vi "PumpValveHeater.vi"() -> ()   [LabVIEW 2015]
uses:
  PumpValve.ctl
  <vilib>/DAQmx/write.llb/DAQmx Write (Digital 1D Bool NChan 1Samp 1Line).vi
  <vilib>/DAQmx/miscellaneous.llb/DAQmx Fill In Error Info.vi
  <vilib>/addons/control/pid/pid.llb/PID (DBL).vi
  <vilib>/addons/control/pid/NI_PID_pid.lvlib
panel:
  out "Numeric 2":dbl
  out "Numeric":dbl
  out "Heater On/off":bool
  out "Meter (Temp Sensor)":dbl(knob) scale=0.0..10.0
  in  "Stop Maintaining Temp":bool
  in  "PID gains Temp":T1={"proportional gain (Kc)"=1.0, "integral time (Ti, min)"=0.01, "derivative time (Td, min)"=0.0} {"derivative time (Td, min)" format="%.3f"; "integral time (Ti, min)" format="%.3f"; "proportional gain (Kc)" format="%.3f"}
  in  "Temp Setting":dbl
  in  "Maintain Temp":bool
  in  "Stop Maintaining Pressure":bool
  in  "PID gains":T1={"proportional gain (Kc)"=1.0, "integral time (Ti, min)"=0.01, "derivative time (Td, min)"=0.0} {"derivative time (Td, min)" format="%.3f"; "integral time (Ti, min)" format="%.3f"; "proportional gain (Kc)" format="%.3f"}
  out "Meter (Pressure Sensor)":dbl(knob) scale=0.0..10.0
  in  "Pressure Setting":dbl
  in  "Maintain pressure":bool
  in  "On/Off Temp":bool
  in  "Manual Mode Temp":bool
  in  "stop controller":bool
  in  "Duty cycle % (0-100)":dbl=50.0
  in  "stop PWM":bool
  in  "Steps in a cycle":i32=256
  in  "Cycle time (s)":dbl=5.0
  in  "On/Off (Pump)":bool
  in  "Open/Close (Blue)":bool
  in  "Open/Close (Green)":bool
  in  "Manual Mode Pump/Valve":bool
  out "Invalid fill%":bool
  out "Tank":u32(slide) scale=0.0..100.0
  in  "Drain %":u32
  in  "Fill %":u32
  in  "Drain":bool
  in  "Stop Program":bool
  in  "Fill":bool
  # "Temp only adjusts up (do nothing to cool?)"
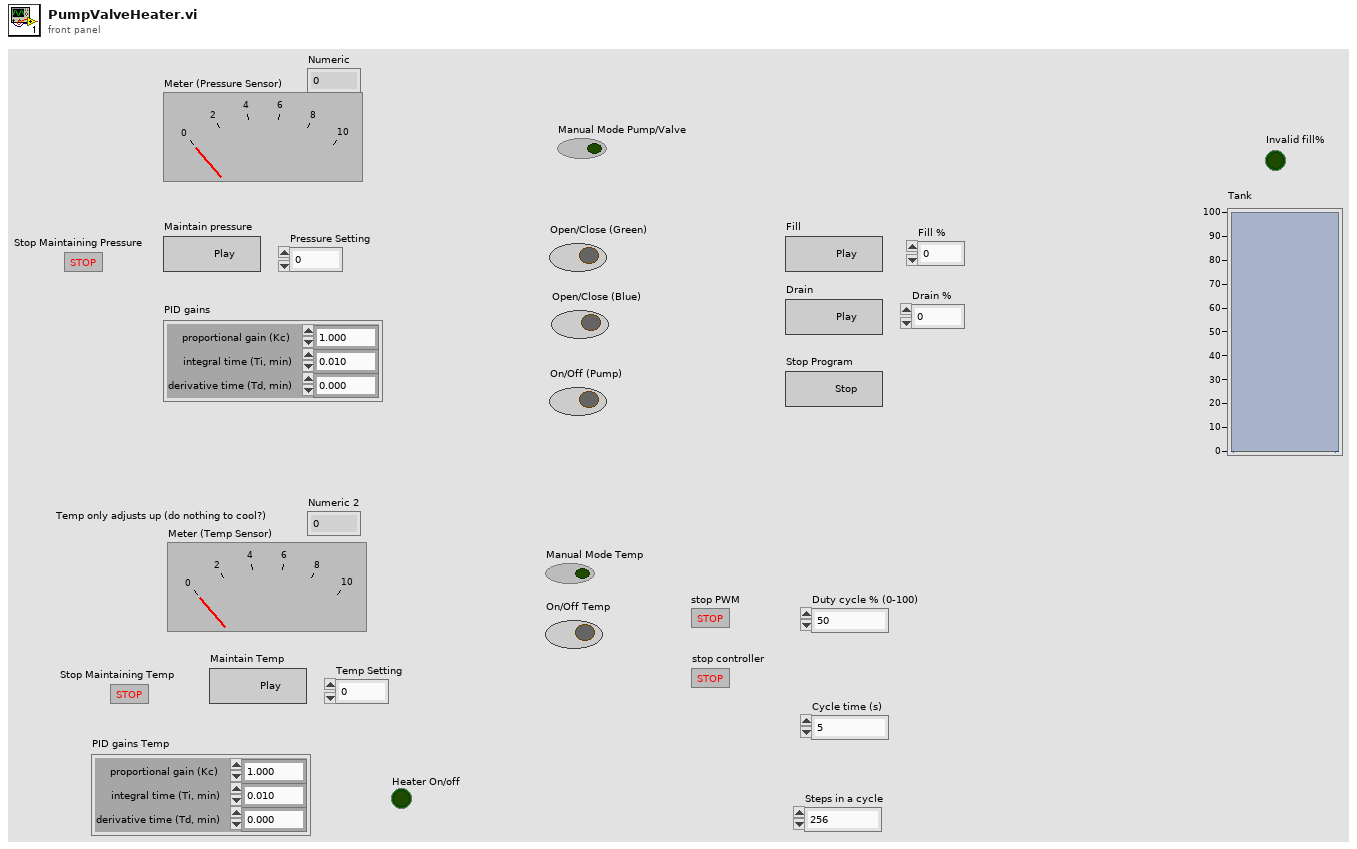
[diagram p1: front panel]
types:
  T1 = cluster{"proportional gain (Kc)":dbl, "integral time (Ti, min)":dbl, "derivative time (Td, min)":dbl}
  T2 = typedef "PumpValve.ctl" = enum16{"PressureSetting", "ManualPressure", "ManualTemp", "Idle Temp", "Set Temp", "Initialize", "Idle", "Fill", "Drain", "Stop"}
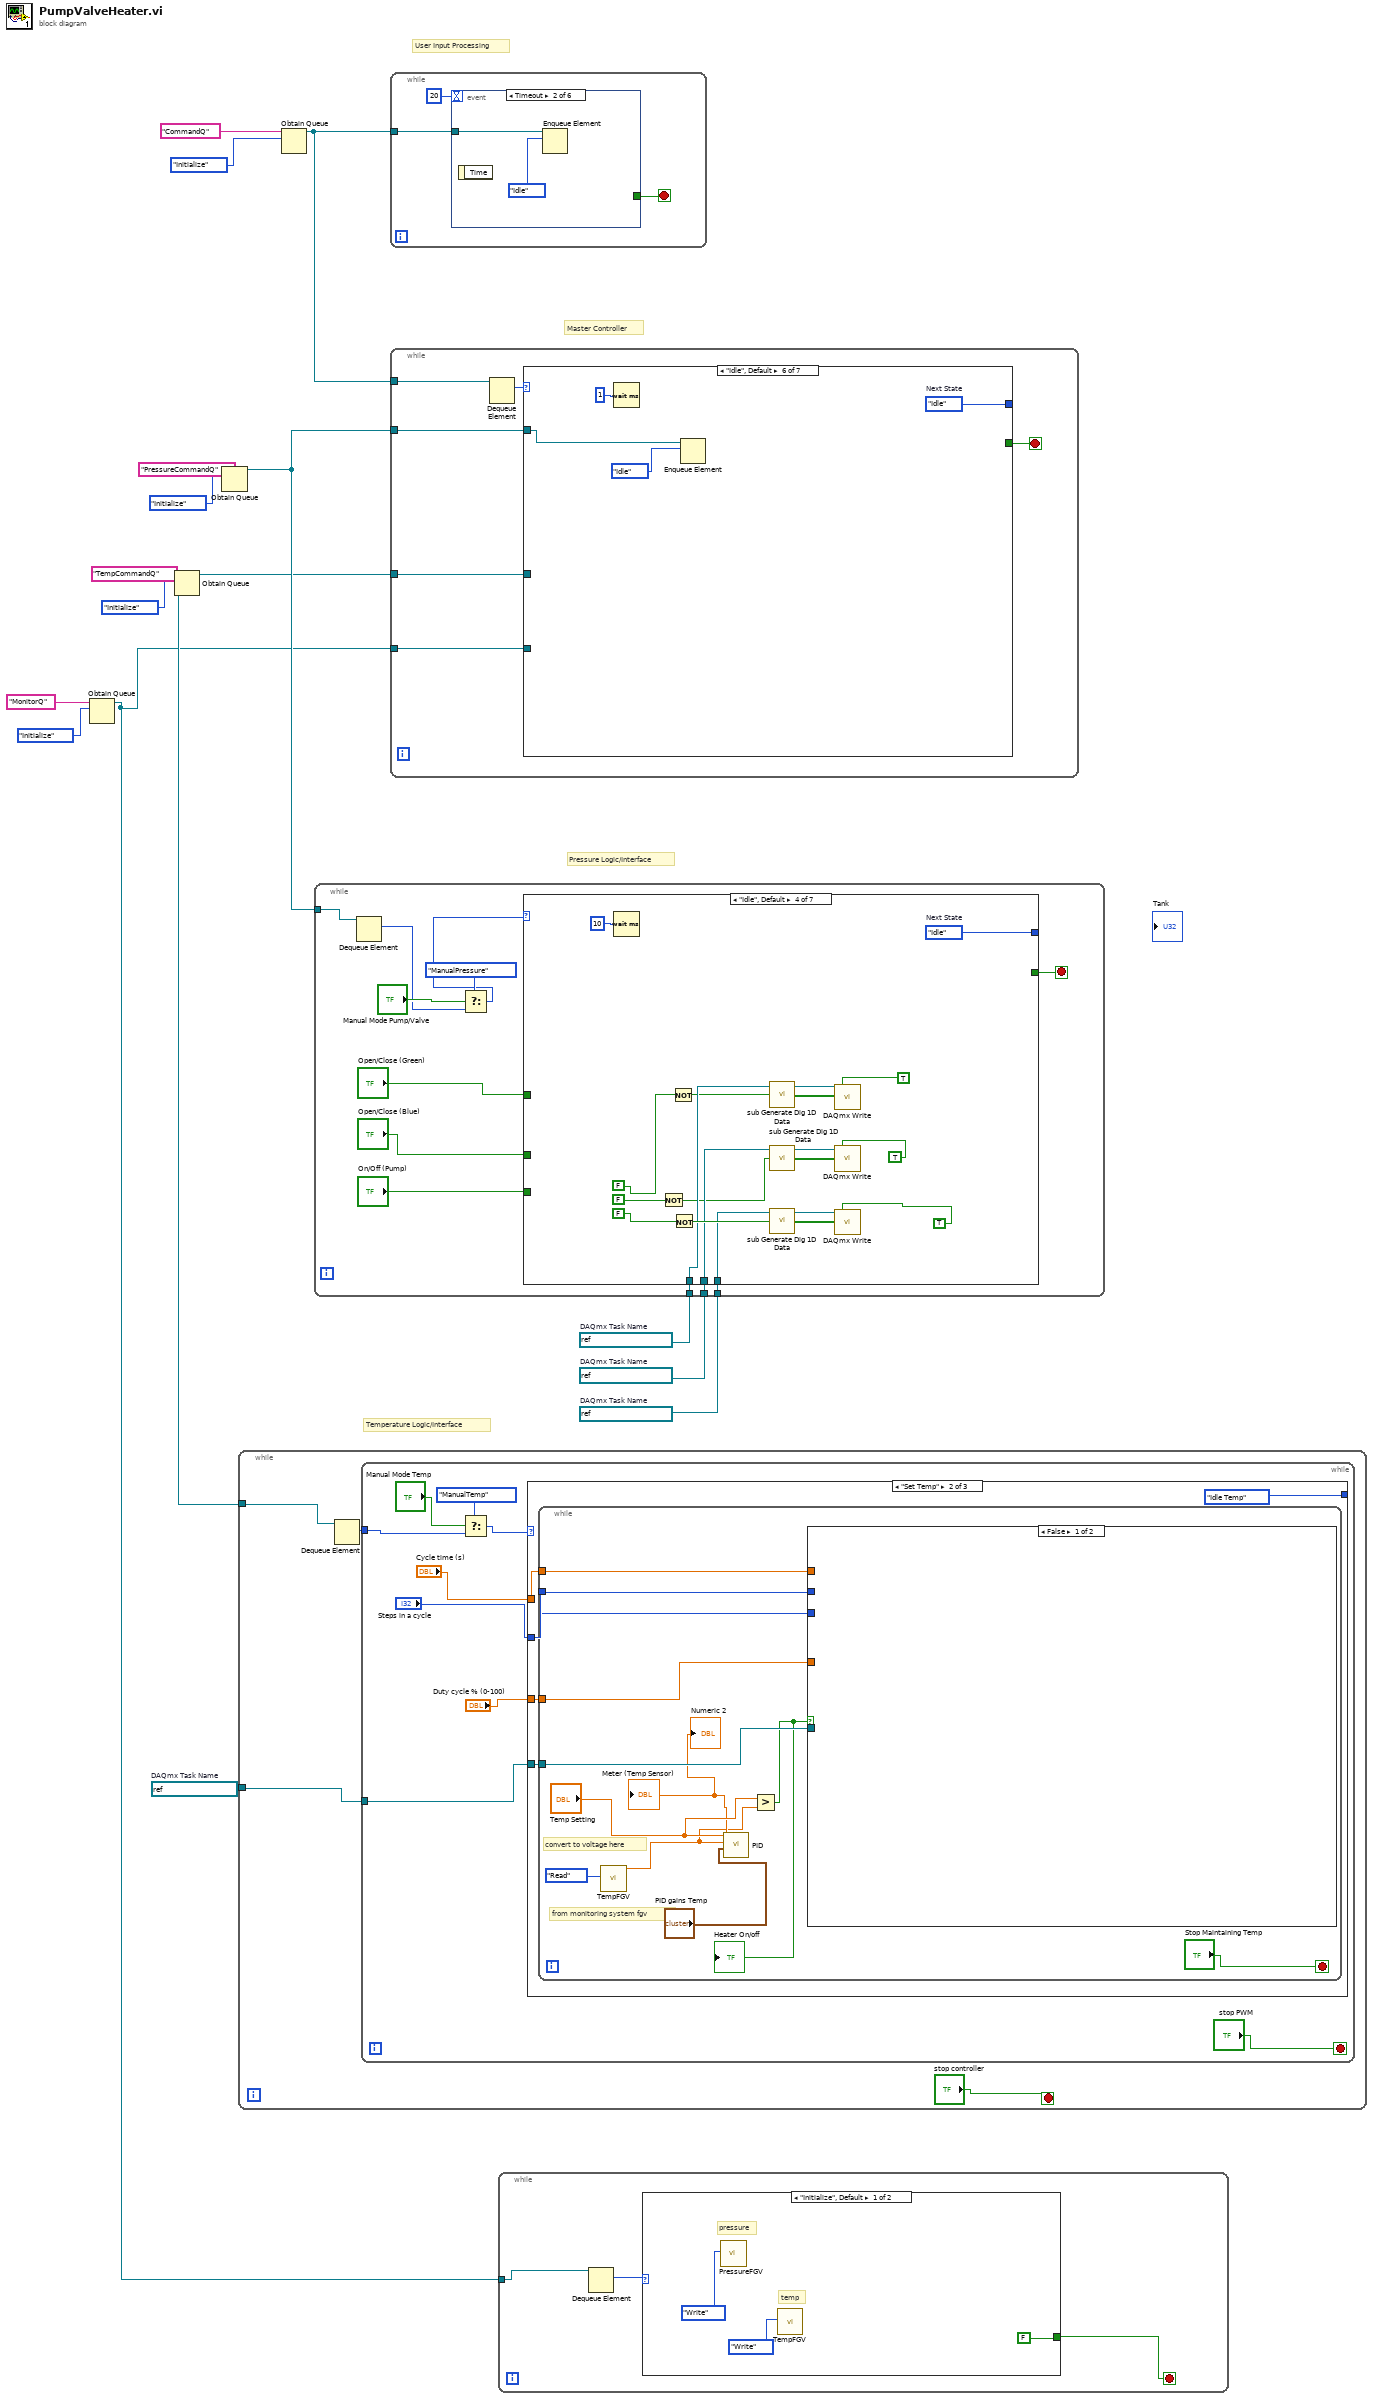
[diagram p0: block diagram]
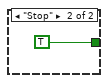
[diagram p2: hidden frame]
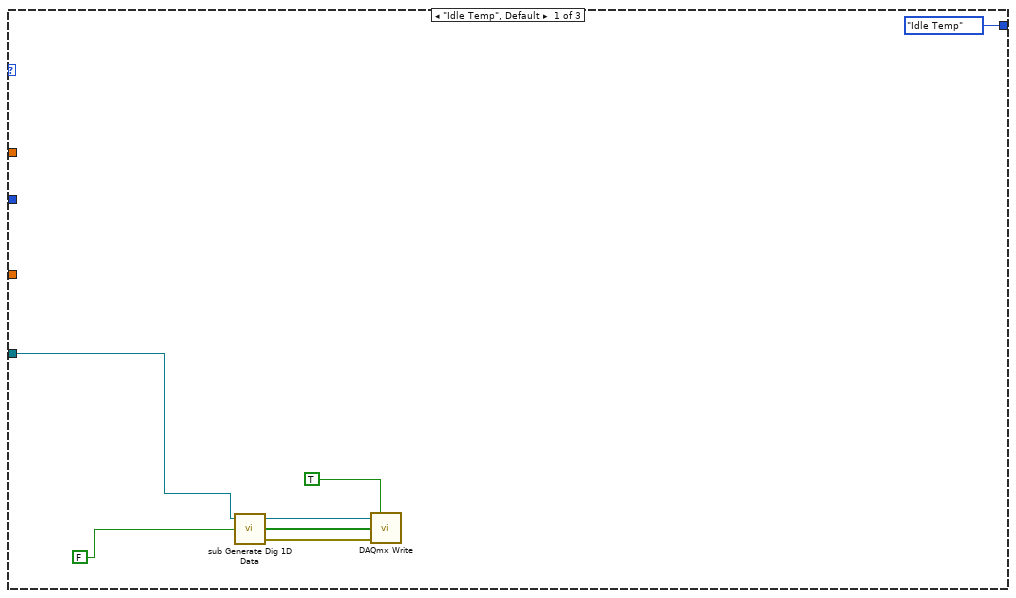
[diagram p3: hidden frame]
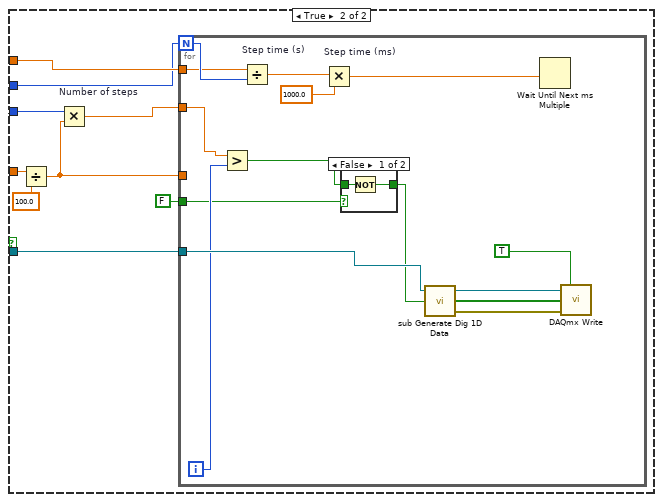
[diagram p4: hidden frame]
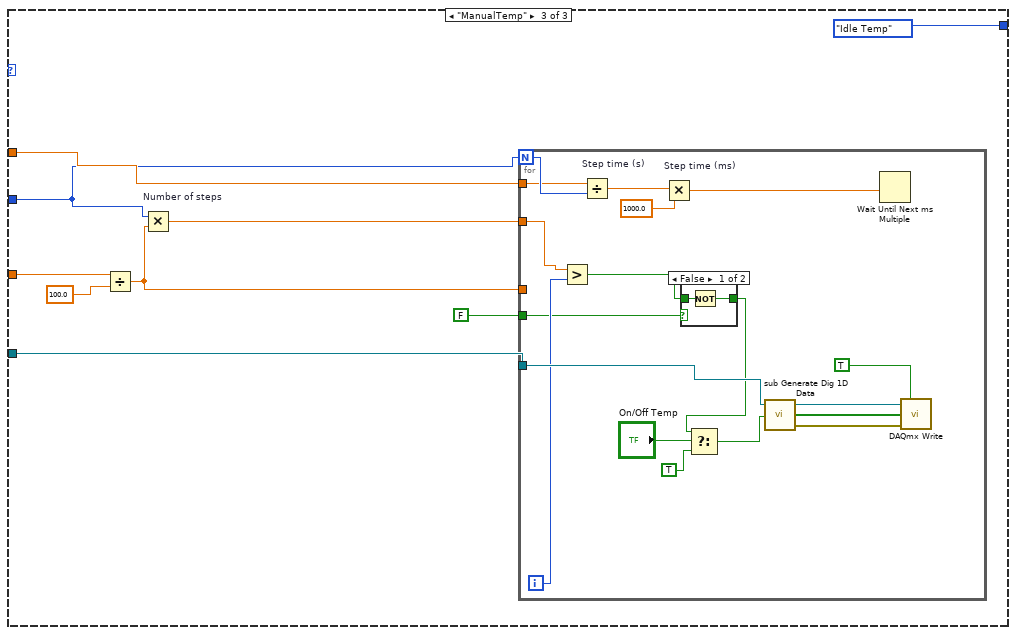
[diagram p6: hidden frame]
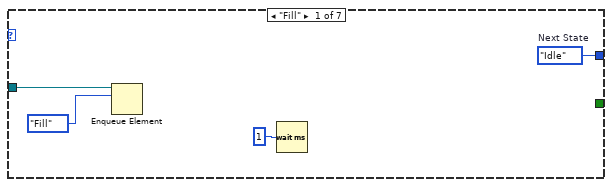
[diagram p8: hidden frame]
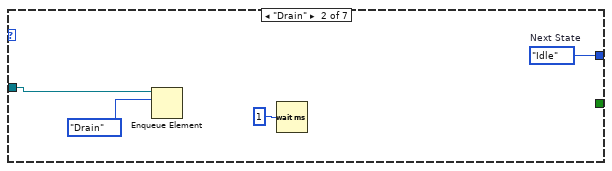
[diagram p9: hidden frame]
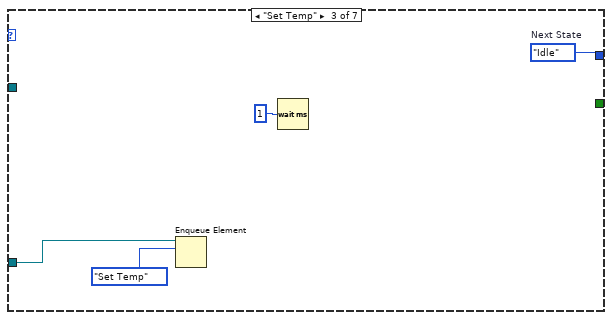
[diagram p10: hidden frame]
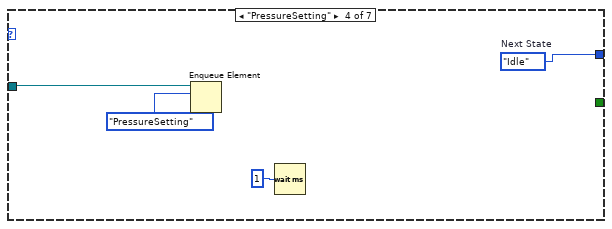
[diagram p11: hidden frame]
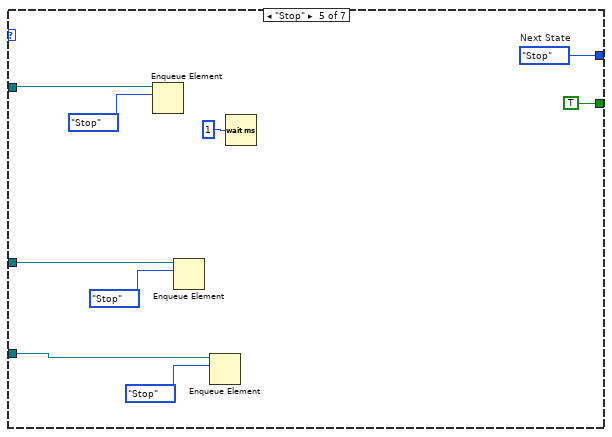
[diagram p12: hidden frame]
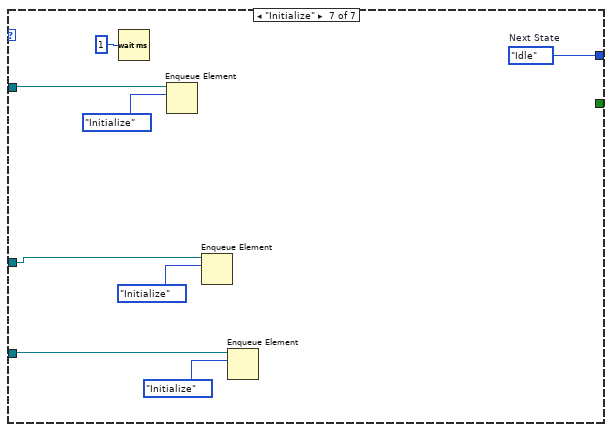
[diagram p13: hidden frame]
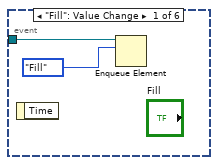
[diagram p14: hidden frame]
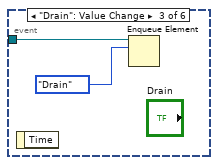
[diagram p15: hidden frame]
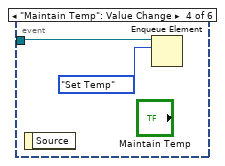
[diagram p16: hidden frame]
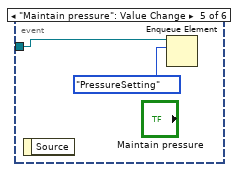
[diagram p17: hidden frame]
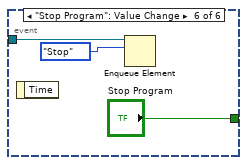
[diagram p18: hidden frame]
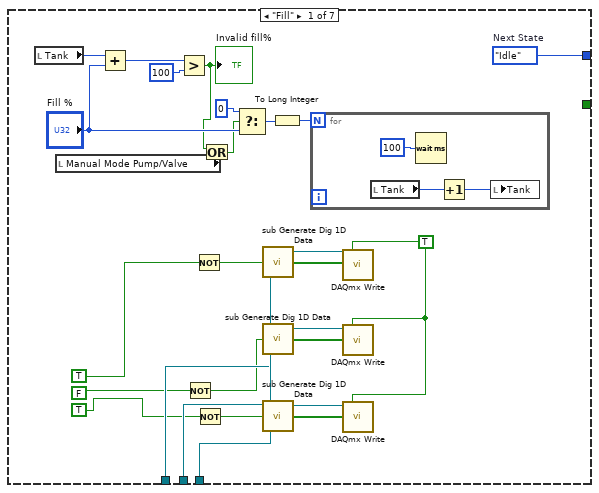
[diagram p19: hidden frame]
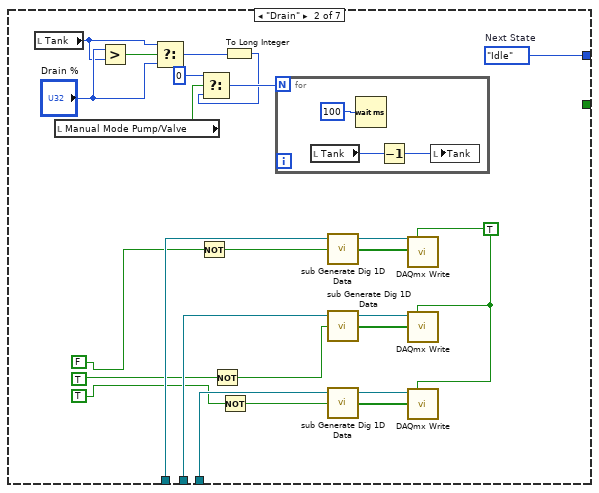
[diagram p20: hidden frame]
diagram:
  w7 = refnum<k21> "DigitalOutBlue"  # DAQmx Task Name
  w12 = refnum<k21> "DigitalOutGreen"  # DAQmx Task Name
  w13 = refnum<k21> "DigitalOutGreen"  # DAQmx Task Name
  w14 = refnum<k21> "DigitalOutGreen"  # DAQmx Task Name
  # "Temperature Logic/Interface"
  # "Pressure Logic/Interface"
  # "Master Controller"
  # "User Input Processing"
  n1 = Obtain Queue(name (unnamed)="MonitorQ", element data type=PumpValve."Initialize" ("States")) -> (queue out=w1:refnum<queue>)  [unwired: 3 in, 2 out]
  n2 = Obtain Queue(name (unnamed)="TempCommandQ", element data type=PumpValve."Initialize" ("States")) -> (queue out=w4:refnum<queue>)  [unwired: 3 in, 2 out]
  n3 = Obtain Queue(name (unnamed)="PressureCommandQ", element data type=PumpValve."Initialize" ("States")) -> (queue out=w8:refnum<queue>)  [unwired: 3 in, 2 out]
  n4 = while {
    tunnel: w7 -> [w20]
    tunnel: w4 -> [w19]
    stop <- "stop controller" stop-if-true
    n5 = Dequeue Element(queue=w19) -> (element=w18:T2)  [unwired: 2 in, 3 out]
    n6 = while {
      tunnel: w20 -> [w29]
      tunnel: w18 -> [w24]
      stop <- "stop PWM" stop-if-true
      n7 = Select(t=PumpValve."ManualTemp", s="Manual Mode Temp", f=w24) -> (s? t:f=w23:T2)
      n8 = case shown="\"Set Temp\"" w23 {
        tunnel: w29 -> [w31 w41 w87]
        tunnel: [PumpValve."Idle Temp" ("States") PumpValve."Idle Temp" ("States") PumpValve."Idle Temp" ("States")] -> _
        tunnel: "Cycle time (s)" -> [_ w39 w81]
        tunnel: "Steps in a cycle" -> [_ w38 w80]
        tunnel: "Duty cycle % (0-100)" -> [_ w37 w79]
        frame "Idle Temp", Default {
          n9 = call <vilib>:"sub Generate Dig 1D Data.vi"("initial value"=FALSE, "task in"=w31) -> ("error out"=w33:errorcluster, "Data"=w34:bool[], "task out"=w35:refnum<k21>)  [unwired: 1 in]
          n10 = call-poly <vilib>:"DAQmx Write.vi"("task/channels in"=w35, "auto start"=TRUE, "data"=w34, "error in"=w33) -> ()  [unwired: 9 in, 3 out]
        }
        frame "Set Temp" {
          n11 = while {
            tunnel: w41 -> [w52]
            tunnel: w39 -> [w51]
            tunnel: w38 -> [w46]
            tunnel: w37 -> [w50]
            stop <- "Stop Maintaining Temp" stop-if-true
            # "convert to voltage here"
            # "from monitoring system fgv"
            n12 = call "TempFGV.vi"("Command"=enum16{"Write", "Read"}."Read") -> ("OUT"=w43:dbl)  [unwired: 10 in]
            n13 = call-poly <vilib>:"PID.vi"("PID gains"="PID gains Temp", "process variable"=w43, "setpoint"="Temp Setting") -> ("output"=→"Meter (Temp Sensor)" →"Numeric 2":dbl)  [unwired: 7 in, 1 out]
            n14 = Greater?(x="Temp Setting", y=w43) -> (0:w45:bool)
            "Heater On/off" <- w45
            n15 = case shown="False" w45 {
              tunnel: w52 -> [_ w60]
              tunnel: w51 -> [_ w55]
              tunnel: w46 -> [_ w54]
              tunnel: w50 -> [_ w53]
              tunnel: w46 -> [_ _]
              frame False {
              }
              frame True {
                n16 = Divide(x=w53, y=100.0) -> (x/y=w58:dbl)
                n17 = Multiply "Number of steps"(x=w54, y=w58) -> (x*y=w57:dbl)
                n18 = for {
                  N: w54 -> [w70]
                  tunnel: w60 -> [w72]
                  tunnel: w58 -> [_]
                  tunnel: w55 -> [w69]
                  tunnel: w57 -> [w65]
                  tunnel: FALSE -> [w62]
                  i -> [w64]
                  n19 = Greater?(x=w65, y=w64) -> (0:w63:bool)
                  n20 = Divide "Step time (s)"(x=w69, y=w70) -> (x/y=w68:dbl)
                  n21 = Multiply "Step time (ms)"(x=w68, y=1000.0) -> (x*y=w66:dbl)
                  n22 = case shown="False" w62 {
                    tunnel: [w76 w78] -> w71
                    tunnel: w63 -> [w77 w78]
                    frame False {
                      n23 = Not(x=w77) -> (.not. x?=w76:bool)
                    }
                    frame True {
                    }
                  }
                  n24 = call <vilib>:"sub Generate Dig 1D Data.vi"("initial value"=w71, "task in"=w72) -> ("error out"=w74:errorcluster, "Data"=w61:bool[], "task out"=w73:refnum<k21>)  [unwired: 1 in]
                  n25 = Wait Until Next ms Multiple(millisecond multiple=w66) -> ()  [unwired: 1 out]
                  n26 = call-poly <vilib>:"DAQmx Write.vi"("task/channels in"=w73, "auto start"=TRUE, "data"=w61, "error in"=w74) -> ()  [unwired: 9 in, 3 out]
                }
              }
            }
          }
        }
        frame "ManualTemp" {
          n27 = Divide(x=w79, y=100.0) -> (x/y=w85:dbl)
          n28 = Multiply "Number of steps"(x=w80, y=w85) -> (x*y=w84:dbl)
          n29 = for {
            N: w80 -> [w100]
            tunnel: w87 -> [w101]
            tunnel: w85 -> [_]
            tunnel: w81 -> [w99]
            tunnel: w84 -> [w95]
            tunnel: FALSE -> [w92]
            i -> [w94]
            n30 = Greater?(x=w95, y=w94) -> (0:w93:bool)
            n31 = Divide "Step time (s)"(x=w99, y=w100) -> (x/y=w98:dbl)
            n32 = Multiply "Step time (ms)"(x=w98, y=1000.0) -> (x*y=w96:dbl)
            n33 = case shown="False" w92 {
              tunnel: [w106 w108] -> w90
              tunnel: w93 -> [w107 w108]
              frame False {
                n34 = Not(x=w107) -> (.not. x?=w106:bool)
              }
              frame True {
              }
            }
            n35 = Select(t=w90, s="On/Off Temp", f=TRUE) -> (s? t:f=w89:bool)
            n36 = call <vilib>:"sub Generate Dig 1D Data.vi"("initial value"=w89, "task in"=w101) -> ("error out"=w104:errorcluster, "Data"=w103:bool[], "task out"=w102:refnum<k21>)  [unwired: 1 in]
            n37 = Wait Until Next ms Multiple(millisecond multiple=w96) -> ()  [unwired: 1 out]
            n38 = call-poly <vilib>:"DAQmx Write.vi"("task/channels in"=w102, "auto start"=TRUE, "data"=w103, "error in"=w104) -> ()  [unwired: 9 in, 3 out]
          }
        }
      }
    }
  }
  n39 = Obtain Queue(name (unnamed)="CommandQ", element data type=PumpValve."Initialize" ("States")) -> (queue out=w11:refnum<queue>)  [unwired: 3 in, 2 out]
  n40 = while {
    tunnel: w8 -> [w120]
    tunnel: w14 -> [w116]
    tunnel: w13 -> [w117]
    tunnel: w12 -> [w118]
    stop <- w119 stop-if-true
    n41 = Dequeue Element(queue=w120) -> (element=w113:T2)  [unwired: 2 in, 3 out]
    n42 = Select(t=PumpValve."ManualPressure", s="Manual Mode Pump/Valve", f=w113) -> (s? t:f=w112:T2)
    n43 = case shown="\"Idle\", Default" w112 {
      tunnel: [w147 w175 w196 w216 w236 w237 w263] -> _
      tunnel: [_ _ w182 _ _ _ _] -> w119
      tunnel: w118 -> [w129 w157 w186 w204 w224 _ w252]
      tunnel: w117 -> [w128 w158 w187 w203 w223 _ w253]
      tunnel: w116 -> [w127 w159 w188 w202 w222 _ w254]
      tunnel: "Open/Close (Green)" -> [_ _ _ _ w219 _ _]
      tunnel: "Open/Close (Blue)" -> [_ _ _ _ w218 _ _]
      tunnel: "On/Off (Pump)" -> [_ _ _ _ w217 _ _]
      frame "Fill" {
        w136 = TRUE
        w147 = PumpValve."Idle"  # Next State
        n44 = local read "Tank"() -> (w146:u32)
        n45 = local read "Manual Mode Pump/Valve"() -> (w138:bool)
        n46 = Add(x=w146, y="Fill %") -> (x+y=w144:u32)
        n47 = Greater?(x=w144, y=u32 100) -> (0:w139:bool)
        "Invalid fill%" <- w139
        n48 = Not(x=FALSE) -> (.not. x?=w124:bool)
        n49 = Not(x=TRUE) -> (.not. x?=w125:bool)
        n50 = Not(x=TRUE) -> (.not. x?=w126:bool)
        n51 = Or(x=w139, y=w138) -> (x .or. y?=w137:bool)
        n52 = Select(t=u32 0, s=w137, f="Fill %") -> (s? t:f=w141:u32)
        n53 = call <vilib>:"sub Generate Dig 1D Data.vi"("initial value"=w125, "task in"=w127) -> ("Data"=w131:bool[], "task out"=w135:refnum<k21>)  [unwired: 1 in, 1 out]
        n54 = call <vilib>:"sub Generate Dig 1D Data.vi"("initial value"=w124, "task in"=w128) -> ("Data"=w132:bool[], "task out"=w134:refnum<k21>)  [unwired: 1 in, 1 out]
        n55 = call <vilib>:"sub Generate Dig 1D Data.vi"("initial value"=w126, "task in"=w129) -> ("Data"=w130:bool[], "task out"=w133:refnum<k21>)  [unwired: 1 in, 1 out]
        n56 = To Long Integer(number=w141) -> (32bit integer=w140:i32)
        n57 = for {
          N: w140 -> [_]
          n58 = local read "Tank"() -> (w150:u32)
          n59 = Wait (ms)(milliseconds to wait=u32 100 ("y")) -> ()  [unwired: 1 out]
          n60 = Increment(x=w150) -> (x+1=w149:u32)
          n61 = local write "Tank"(w149) -> ()
        }
        n62 = call-poly <vilib>:"DAQmx Write.vi"("task/channels in"=w135, "auto start"=w136, "data"=w131) -> ()  [unwired: 10 in, 3 out]
        n63 = call-poly <vilib>:"DAQmx Write.vi"("task/channels in"=w134, "auto start"=w136, "data"=w132) -> ()  [unwired: 10 in, 3 out]
        n64 = call-poly <vilib>:"DAQmx Write.vi"("task/channels in"=w133, "auto start"=w136, "data"=w130) -> ()  [unwired: 10 in, 3 out]
      }
      frame "Drain" {
        w160 = TRUE
        w175 = PumpValve."Idle"  # Next State
        n65 = local read "Tank"() -> (w172:u32)
        n66 = local read "Manual Mode Pump/Valve"() -> (w170:bool)
        n67 = Greater?(x="Drain %", y=w172) -> (0:w171:bool)
        n68 = Select(t=w172, s=w171, f="Drain %") -> (s? t:f=w174:u32)
        n69 = Not(x=FALSE) -> (.not. x?=w155:bool)
        n70 = Not(x=TRUE) -> (.not. x?=w154:bool)
        n71 = Not(x=TRUE) -> (.not. x?=w156:bool)
        n72 = To Long Integer(number=w174) -> (32bit integer=w167:i32)
        n73 = Select(t=0, s=w170, f=w167) -> (s? t:f=w168:i32)
        n74 = for {
          N: w168 -> [_]
          n75 = local read "Tank"() -> (w177:u32)
          n76 = Wait (ms)(milliseconds to wait=u32 100) -> ()  [unwired: 1 out]
          n77 = Decrement(x=w177) -> (x-1=w178:u32)
          n78 = local write "Tank"(w178) -> ()
        }
        n79 = call <vilib>:"sub Generate Dig 1D Data.vi"("initial value"=w155, "task in"=w159) -> ("Data"=w165:bool[], "task out"=w161:refnum<k21>)  [unwired: 1 in, 1 out]
        n80 = call <vilib>:"sub Generate Dig 1D Data.vi"("initial value"=w154, "task in"=w158) -> ("Data"=w164:bool[], "task out"=w162:refnum<k21>)  [unwired: 1 in, 1 out]
        n81 = call <vilib>:"sub Generate Dig 1D Data.vi"("initial value"=w156, "task in"=w157) -> ("Data"=w166:bool[], "task out"=w163:refnum<k21>)  [unwired: 1 in, 1 out]
        n82 = call-poly <vilib>:"DAQmx Write.vi"("task/channels in"=w161, "auto start"=w160, "data"=w165) -> ()  [unwired: 10 in, 3 out]
        n83 = call-poly <vilib>:"DAQmx Write.vi"("task/channels in"=w162, "auto start"=w160, "data"=w164) -> ()  [unwired: 10 in, 3 out]
        n84 = call-poly <vilib>:"DAQmx Write.vi"("task/channels in"=w163, "auto start"=w160, "data"=w166) -> ()  [unwired: 10 in, 3 out]
      }
      frame "Stop" {
        w195 = TRUE
        w182 = TRUE  # Off
        w196 = PumpValve."Stop"  # Next State
        n85 = Not(x=FALSE) -> (.not. x?=w183:bool)
        n86 = Not(x=FALSE) -> (.not. x?=w184:bool)
        n87 = Not(x=FALSE) -> (.not. x?=w185:bool)
        n88 = call <vilib>:"sub Generate Dig 1D Data.vi"("initial value"=w184, "task in"=w188) -> ("Data"=w190:bool[], "task out"=w194:refnum<k21>)  [unwired: 1 in, 1 out]
        n89 = call <vilib>:"sub Generate Dig 1D Data.vi"("initial value"=w183, "task in"=w187) -> ("Data"=w191:bool[], "task out"=w193:refnum<k21>)  [unwired: 1 in, 1 out]
        n90 = call <vilib>:"sub Generate Dig 1D Data.vi"("initial value"=w185, "task in"=w186) -> ("Data"=w189:bool[], "task out"=w192:refnum<k21>)  [unwired: 1 in, 1 out]
        n91 = call-poly <vilib>:"DAQmx Write.vi"("task/channels in"=w194, "auto start"=w195, "data"=w190) -> ()  [unwired: 10 in, 3 out]
        n92 = call-poly <vilib>:"DAQmx Write.vi"("task/channels in"=w193, "auto start"=w195, "data"=w191) -> ()  [unwired: 10 in, 3 out]
        n93 = call-poly <vilib>:"DAQmx Write.vi"("task/channels in"=w192, "auto start"=w195, "data"=w189) -> ()  [unwired: 10 in, 3 out]
      }
      frame "Idle", Default {
        w216 = PumpValve."Idle"  # Next State
        n94 = Wait (ms)(milliseconds to wait=u32 10) -> ()  [unwired: 1 out]
        n95 = Not(x=FALSE) -> (.not. x?=w200:bool)
        n96 = Not(x=FALSE) -> (.not. x?=w201:bool)
        n97 = Not(x=FALSE) -> (.not. x?=w207:bool)
        n98 = call <vilib>:"sub Generate Dig 1D Data.vi"("initial value"=w201, "task in"=w202) -> ("Data"=w209:bool[], "task out"=w213:refnum<k21>)  [unwired: 1 in, 1 out]
        n99 = call <vilib>:"sub Generate Dig 1D Data.vi"("initial value"=w200, "task in"=w203) -> ("Data"=w210:bool[], "task out"=w212:refnum<k21>)  [unwired: 1 in, 1 out]
        n100 = call <vilib>:"sub Generate Dig 1D Data.vi"("initial value"=w207, "task in"=w204) -> ("Data"=w208:bool[], "task out"=w211:refnum<k21>)  [unwired: 1 in, 1 out]
        n101 = call-poly <vilib>:"DAQmx Write.vi"("task/channels in"=w213, "auto start"=TRUE, "data"=w209) -> ()  [unwired: 10 in, 3 out]
        n102 = call-poly <vilib>:"DAQmx Write.vi"("task/channels in"=w212, "auto start"=TRUE, "data"=w210) -> ()  [unwired: 10 in, 3 out]
        n103 = call-poly <vilib>:"DAQmx Write.vi"("task/channels in"=w211, "auto start"=TRUE, "data"=w208) -> ()  [unwired: 10 in, 3 out]
      }
      frame "ManualPressure" {
        w236 = PumpValve."Idle"  # Next State
        n104 = Wait (ms)(milliseconds to wait=u32 10) -> ()  [unwired: 1 out]
        n105 = Not(x=w218) -> (.not. x?=w220:bool)
        n106 = Not(x=w219) -> (.not. x?=w221:bool)
        n107 = Not(x=w217) -> (.not. x?=w227:bool)
        n108 = call <vilib>:"sub Generate Dig 1D Data.vi"("initial value"=w221, "task in"=w222) -> ("Data"=w229:bool[], "task out"=w233:refnum<k21>)  [unwired: 1 in, 1 out]
        n109 = call <vilib>:"sub Generate Dig 1D Data.vi"("initial value"=w220, "task in"=w223) -> ("Data"=w230:bool[], "task out"=w232:refnum<k21>)  [unwired: 1 in, 1 out]
        n110 = call <vilib>:"sub Generate Dig 1D Data.vi"("initial value"=w227, "task in"=w224) -> ("Data"=w228:bool[], "task out"=w231:refnum<k21>)  [unwired: 1 in, 1 out]
        n111 = call-poly <vilib>:"DAQmx Write.vi"("task/channels in"=w233, "auto start"=TRUE, "data"=w229) -> ()  [unwired: 10 in, 3 out]
        n112 = call-poly <vilib>:"DAQmx Write.vi"("task/channels in"=w232, "auto start"=TRUE, "data"=w230) -> ()  [unwired: 10 in, 3 out]
        n113 = call-poly <vilib>:"DAQmx Write.vi"("task/channels in"=w231, "auto start"=TRUE, "data"=w228) -> ()  [unwired: 10 in, 3 out]
      }
      frame "PressureSetting" {
        w237 = PumpValve."Idle"  # Next State
        n114 = while {
          stop <- "Stop Maintaining Pressure" stop-if-true
          # "from monitoring system"
          # "output to hardware"
          n115 = call "PressureFGV.vi"("IN"=enum16{"Write", "Read"}."Read" ("Command")) -> ("OUT"=w239:dbl)  [unwired: 10 in]
          n116 = call-poly <vilib>:"PID.vi"("PID gains"="PID gains", "process variable"=w239, "setpoint"="Pressure Setting") -> ("output"=→"Meter (Pressure Sensor)" →"Numeric":dbl)  [unwired: 7 in, 1 out]
        }
      }
      frame "Initialize" {
        w263 = PumpValve."Idle"  # Next State
        n117 = Wait (ms)(milliseconds to wait=u32 1) -> ()  [unwired: 1 out]
        n118 = Not(x=FALSE) -> (.not. x?=w248:bool)
        n119 = Not(x=FALSE) -> (.not. x?=w247:bool)
        n120 = Not(x=FALSE) -> (.not. x?=w251:bool)
        n121 = call <vilib>:"sub Generate Dig 1D Data.vi"("initial value"=w248, "task in"=w254) -> ("Data"=w256:bool[], "task out"=w260:refnum<k21>)  [unwired: 1 in, 1 out]
        n122 = call <vilib>:"sub Generate Dig 1D Data.vi"("initial value"=w247, "task in"=w253) -> ("Data"=w257:bool[], "task out"=w259:refnum<k21>)  [unwired: 1 in, 1 out]
        n123 = call <vilib>:"sub Generate Dig 1D Data.vi"("initial value"=w251, "task in"=w252) -> ("Data"=w255:bool[], "task out"=w258:refnum<k21>)  [unwired: 1 in, 1 out]
        n124 = call-poly <vilib>:"DAQmx Write.vi"("task/channels in"=w260, "auto start"=TRUE, "data"=w256) -> ()  [unwired: 10 in, 3 out]
        n125 = call-poly <vilib>:"DAQmx Write.vi"("task/channels in"=w259, "auto start"=TRUE, "data"=w257) -> ()  [unwired: 10 in, 3 out]
        n126 = call-poly <vilib>:"DAQmx Write.vi"("task/channels in"=w258, "auto start"=TRUE, "data"=w255) -> ()  [unwired: 10 in, 3 out]
      }
    }
  }
  n127 = while {
    tunnel: w11 -> [w265]
    stop <- w264 stop-if-true
    n128 = event shown="[1] Timeout" {
      selector: _ -> [_ _ _ _ _ _]
      dyn-events: _ -> [_ _ _ _ _ _]
      timeout: 20 -> [_ _ _ _ _ _]
      tunnel: w265 -> [w268 w270 w272 w273 w276 w279]
      tunnel: [_ _ _ _ _ "Stop Program"] -> w264
      event "Fill": Value Change {
        n129 = event-data() -> ()  [unwired: 1 in, 1 out]
        n130 = Enqueue Element(queue=w268, element=PumpValve."Fill" ("States")) -> ()  [unwired: 2 in, 3 out]
      }
      event Timeout {
        n131 = event-data() -> ()  [unwired: 1 in, 1 out]
        n132 = Enqueue Element(queue=w270, element=PumpValve."Idle" ("States")) -> ()  [unwired: 2 in, 3 out]
      }
      event "Drain": Value Change {
        n133 = event-data() -> ()  [unwired: 1 in, 1 out]
        n134 = Enqueue Element(queue=w272, element=PumpValve."Drain" ("States")) -> ()  [unwired: 2 in, 3 out]
      }
      event "Maintain Temp": Value Change {
        n135 = event-data() -> ()  [unwired: 1 in, 1 out]
        n136 = Enqueue Element(queue=w273, element=PumpValve."Set Temp" ("States")) -> ()  [unwired: 2 in, 3 out]
      }
      event "Maintain pressure": Value Change {
        n137 = event-data() -> ()  [unwired: 1 in, 1 out]
        n138 = Enqueue Element(queue=w276, element=PumpValve."PressureSetting" ("States")) -> ()  [unwired: 2 in, 3 out]
      }
      event "Stop Program": Value Change {
        n139 = event-data() -> ()  [unwired: 1 in, 1 out]
        n140 = Enqueue Element(queue=w279, element=PumpValve."Stop" ("States")) -> ()  [unwired: 2 in, 3 out]
      }
    }
  }
  n141 = while {
    tunnel: w11 -> [w284]
    tunnel: w8 -> [w283]
    tunnel: w4 -> [w281]
    tunnel: w1 -> [w280]
    stop <- w282 stop-if-true
    n142 = Dequeue Element(queue=w284) -> (element=w285:T2)  [unwired: 2 in, 3 out]
    n143 = case shown="\"Idle\", Default" w285 {
      tunnel: [w289 w293 w295 w299 w310 w314 w322] -> _
      tunnel: w283 -> [w286 w290 _ w298 w307 w311 w319]
      tunnel: [_ _ _ _ TRUE _ _] -> w282
      tunnel: w281 -> [_ _ w294 _ w304 _ w316]
      tunnel: w280 -> [_ _ _ _ w302 _ w315]
      frame "Fill" {
        w289 = PumpValve."Idle"  # Next State
        n144 = Enqueue Element(queue=w286, element=PumpValve."Fill" ("States")) -> ()  [unwired: 2 in, 3 out]
        n145 = Wait (ms)(milliseconds to wait=u32 1) -> ()  [unwired: 1 out]
      }
      frame "Drain" {
        w293 = PumpValve."Idle"  # Next State
        n146 = Enqueue Element(queue=w290, element=PumpValve."Drain" ("States")) -> ()  [unwired: 2 in, 3 out]
        n147 = Wait (ms)(milliseconds to wait=u32 1) -> ()  [unwired: 1 out]
      }
      frame "Set Temp" {
        w295 = PumpValve."Idle"  # Next State
        n148 = Enqueue Element(queue=w294, element=PumpValve."Set Temp" ("States")) -> ()  [unwired: 2 in, 3 out]
        n149 = Wait (ms)(milliseconds to wait=u32 1) -> ()  [unwired: 1 out]
      }
      frame "PressureSetting" {
        w299 = PumpValve."Idle"  # Next State
        n150 = Enqueue Element(queue=w298, element=PumpValve."PressureSetting" ("States")) -> ()  [unwired: 2 in, 3 out]
        n151 = Wait (ms)(milliseconds to wait=u32 1) -> ()  [unwired: 1 out]
      }
      frame "Stop" {
        w310 = PumpValve."Stop"  # Next State
        n152 = Enqueue Element(queue=w307, element=PumpValve."Stop" ("States")) -> ()  [unwired: 2 in, 3 out]
        n153 = Enqueue Element(queue=w304, element=PumpValve."Stop" ("States")) -> ()  [unwired: 2 in, 3 out]
        n154 = Enqueue Element(queue=w302, element=PumpValve."Stop" ("States")) -> ()  [unwired: 2 in, 3 out]
        n155 = Wait (ms)(milliseconds to wait=u32 1) -> ()  [unwired: 1 out]
      }
      frame "Idle", Default {
        w314 = PumpValve."Idle"  # Next State
        n156 = Wait (ms)(milliseconds to wait=u32 1) -> ()  [unwired: 1 out]
        n157 = Enqueue Element(queue=w311, element=PumpValve."Idle" ("States")) -> ()  [unwired: 2 in, 3 out]
      }
      frame "Initialize" {
        w322 = PumpValve."Idle"  # Next State
        n158 = Wait (ms)(milliseconds to wait=u32 1) -> ()  [unwired: 1 out]
        n159 = Enqueue Element(queue=w319, element=PumpValve."Initialize" ("States")) -> ()  [unwired: 2 in, 3 out]
        n160 = Enqueue Element(queue=w316, element=PumpValve."Initialize" ("States")) -> ()  [unwired: 2 in, 3 out]
        n161 = Enqueue Element(queue=w315, element=PumpValve."Initialize" ("States")) -> ()  [unwired: 2 in, 3 out]
      }
    }
  }
  n162 = while {
    tunnel: w1 -> [w325]
    stop <- w323 stop-if-true
    n163 = Dequeue Element(queue=w325) -> (element=w324:T2)  [unwired: 2 in, 3 out]
    n164 = case shown="\"Initialize\", Default" w324 {
      tunnel: [FALSE TRUE] -> w323
      frame "Initialize", Default {
        # "temp"
        # "pressure"
        n165 = call "PressureFGV.vi"("Command"=enum16{"Write", "Read"}."Write") -> ()  [unwired: 10 in, 1 out]
        n166 = call "TempFGV.vi"("Command"=enum16{"Write", "Read"}."Write") -> ()  [unwired: 10 in, 1 out]
      }
      frame "Stop" {
      }
    }
  }
